vi "String.Replace if Empty.vi"(10 "New":string, 11 "Old":string) -> (3 "Updated":string)   [LabVIEW 2019]
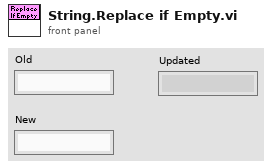
[diagram p1: front panel]
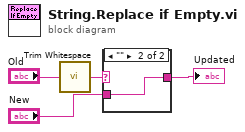
[diagram p0: block diagram]
diagram:
  n1 = call <vilib>:"Trim Whitespace.vi"("string"="Old") -> ("trimmed string"=w4:string)  [unwired: 1 in]
  n2 = case shown="\"\"" w4 {
    selector: w4 -> [w5 _]
    tunnel: [w5 w6] -> w1
    tunnel: "New" -> [_ w6]
    frame Default {
    }
    frame "" {
    }
  }
  "Updated" <- w1
